vi "Get ID.vi"(8 "error in (no error)":errorcluster) -> (0 "error out":errorcluster, 3 "ID":string)   [LabVIEW 2011]
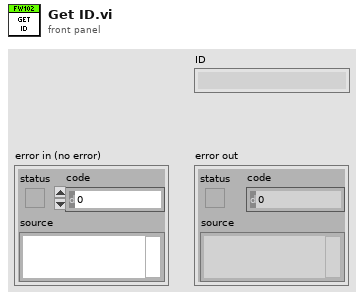
[diagram p1: front panel]
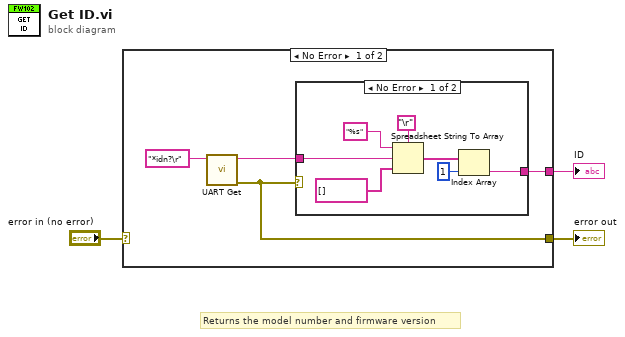
[diagram p0: block diagram]
diagram:
  # "Returns the model number and firmware version"
  n1 = case shown="No Error" "error in (no error)" {
    selector: "error in (no error)" -> [_ w15]
    tunnel: [w7 _] -> w3
    tunnel: [w4 w15] -> w2
    frame No Error {
      n2 = call "UART Get.vi"("Command"="*idn?\r" ("Input Command String")) -> ("error out"=w4:errorcluster, "Returned String"=w5:string)  [unwired: 9 in]
      n3 = case shown="No Error" w4 {
        tunnel: w5 -> [w14 _]
        tunnel: [w8 _] -> w7
        frame No Error {
          n4 = Spreadsheet String To Array(delimiter (Tab)="\r", format string="%s", spreadsheet string=w14, array type (2D Dbl)=string[] []) -> (array=w10:string[])
          n5 = Index Array(array=w10, index=1) -> (element=w8:string)
        }
        frame Error {
        }
      }
    }
    frame Error {
    }
  }
  "ID" <- w3
  "error out" <- w2
